vi "P541 Test.vi"() -> ()   [LabVIEW 2014]
uses:
  Controls/StageStates.ctl
panel:
  out "x-y":u32
  in  "Abort":refnum<vi>
  in  "stop":bool
  out "Monitor":cluster{"Numeric":dbl}(graph) caption="N664"
  in  "Sample Z - P541":T1={"Step Up"=FALSE, "Step Down"=FALSE, "Z Position"=0.0, "Step Size (um)"=1.0}
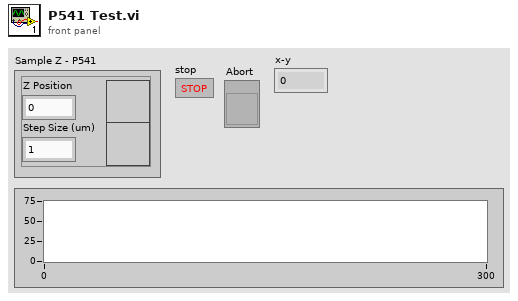
[diagram p1: front panel]
types:
  T1 = cluster{"Step Up":bool, "Step Down":bool, "Z Position":dbl, "Step Size (um)":dbl}
  T2 = typedef "StageStates.ctl" = enum16{"POSITION", "MVR", "MOVE", "HALT", "ONTARGET", "ERROR", "EXIT", "HOME", "ZEROPOS", "NANOPOS", "QUIT", "ANALOG"}
  T3 = cluster{"Step Up":bool, "Step Down":bool, "Z Position":bool, "Step Size (um)":bool}
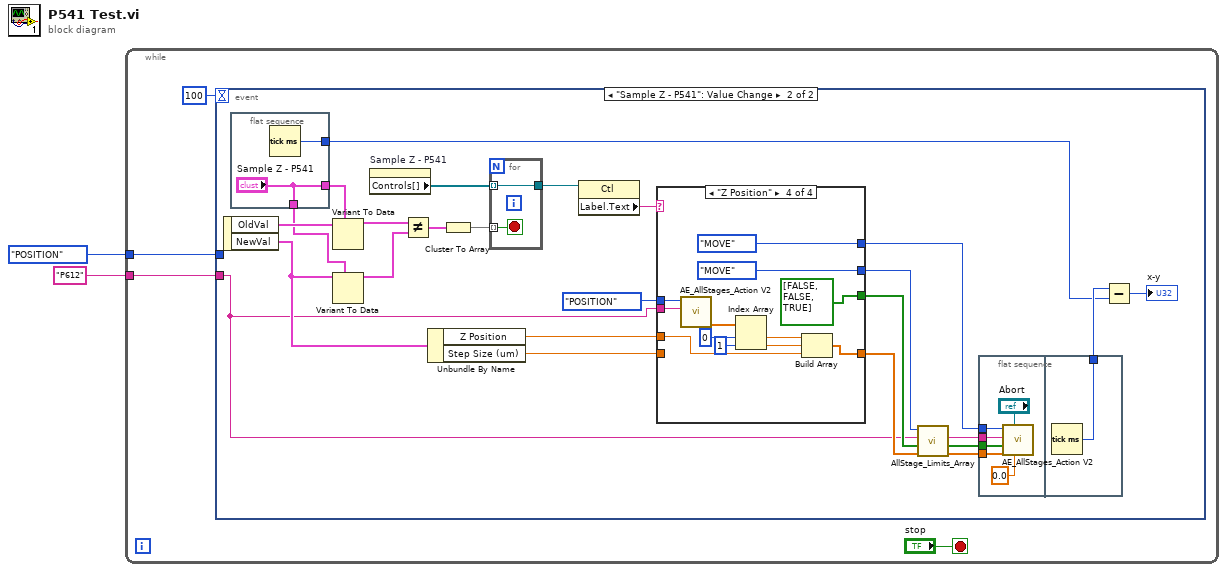
[diagram p0: block diagram]
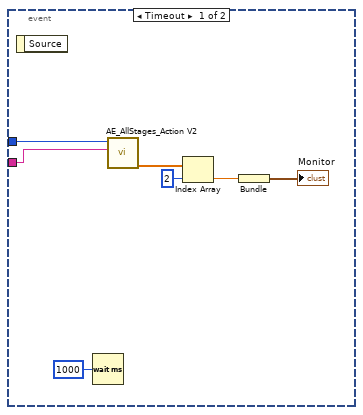
[diagram p2: hidden frame]
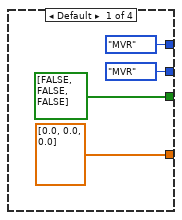
[diagram p3: hidden frame]
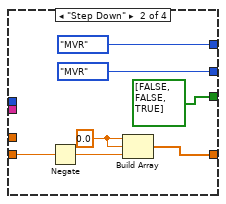
[diagram p4: hidden frame]
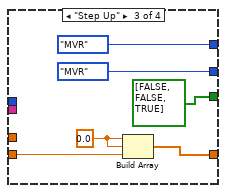
[diagram p5: hidden frame]
diagram:
  n1 = while {
    tunnel: StageStates."POSITION" ("Action") -> [w5]
    tunnel: "P612" ("Stage ID") -> [w4]
    stop <- "stop" stop-if-true
    n2 = event shown="[1] \"Sample Z - P541\": Value Change" {
      selector: _ -> [_ _]
      dyn-events: _ -> [_ _]
      timeout: 100 -> [_ _]
      tunnel: w5 -> [w12 _]
      tunnel: w4 -> [w11 w18]
      event Timeout {
        n3 = event-data() -> ()  [unwired: 1 in, 1 out]
        n4 = Wait (ms)(milliseconds to wait=u32 1000) -> ()  [unwired: 1 out]
        n5 = call "AE_AllStages_Action V2.vi"("Stage ID"=w11, "Action"=w12) -> ("Position Out"=w10:dbl[])  [unwired: 7 in, 2 out]
        n6 = Index Array(array=w10, index=2) -> (element=w8:dbl)
        n7 = Bundle("Numeric"=w8) -> (→"Monitor":cluster{"Numeric":dbl})  [unwired: 1 in]
      }
      event "Sample Z - P541": Value Change {
        n8 = event-data() -> ("OldVal"=w38:T1, "NewVal"=w29:T1)  [unwired: 1 in]
        n9 = flat-sequence {
          tunnel: ["Sample Z - P541"] -> w36
          tunnel: ["Sample Z - P541"] -> w17
          tunnel: [w39] -> w15
          frame #0 {
            n10 = Tick Count (ms)() -> (millisecond timer value=w39:u32)
          }
        }
        n11 = Variant To Data(type=w36, Variant=w38) -> (data=w37:T1)  [unwired: 1 in, 1 out]
        n12 = Variant To Data(type=w17, Variant=w29) -> (data=w35:T1)  [unwired: 1 in, 1 out]
        n13 = property on="Sample Z - P541" class="Clust"() -> ("Controls[]"=w32:refnum<vi>[])  [unwired: 2 in, 2 out]
        n14 = Not Equal?(x=w37, y=w35) -> (x != y?=w34:T3)
        n15 = Unbundle By Name(w29) -> ("Z Position"=w27:dbl, "Step Size (um)"=w28:dbl)
        n16 = Cluster To Array(cluster=w34) -> (array=w33:bool[])
        n17 = for {
          tunnel: w33 -> [w77] mode=indexing
          tunnel: w32 -> [w78] mode=indexing
          tunnel: [w78] -> w31
          stop <- w77 stop-if-true
        }
        n18 = property class="Ctl"(reference=w31) -> ("Label.Text"=w30:string)  [unwired: 1 in, 2 out]
        n19 = case shown="\"Z Position\"" w30 {
          tunnel: w28 -> [_ w55 w59 _]
          tunnel: [StageStates."MVR" ("Action") StageStates."MVR" ("Action") StageStates."MVR" ("Action") StageStates."MOVE" ("Action")] -> w25
          tunnel: [enum16{"MOVE", "MVR"}."MVR" ("MOVE/MVR") enum16{"MOVE", "MVR"}."MVR" ("MOVE/MVR") enum16{"MOVE", "MVR"}."MVR" ("MOVE/MVR") enum16{"MOVE", "MVR"}."MOVE" ("MOVE/MVR")] -> w26
          tunnel: [bool[] [FALSE, FALSE, FALSE] bool[] [FALSE, FALSE, TRUE] bool[] [FALSE, FALSE, TRUE] bool[] [FALSE, FALSE, TRUE]] -> w20
          tunnel: [dbl[] [0.0, 0.0, 0.0] w54 w61 w73] -> w21
          tunnel: w27 -> [_ _ _ w65]
          tunnel: StageStates."POSITION" ("Action") -> [_ _ _ w72]
          tunnel: w18 -> [_ _ _ w71]
          frame Default {
          }
          frame "Step Down" {
            w52 = 0.0 ("element")
            n20 = Negate(x=w55) -> (-x=w53:dbl)
            n21 = Build Array(w52, w52, w53) -> (w54:dbl[])
          }
          frame "Step Up" {
            w60 = 0.0 ("element")
            n22 = Build Array(w60, w60, w59) -> (w61:dbl[])
          }
          frame "Z Position" {
            n23 = call "AE_AllStages_Action V2.vi"("Stage ID"=w71, "Action"=w72) -> ("Position Out"=w70:dbl[])  [unwired: 7 in, 2 out]
            n24 = Index Array(array=w70, index #1=0 ("index"), index #2=1 ("index")) -> (element #1=w67:dbl, element #2=w66:dbl)
            n25 = Build Array(w67, w66, w65) -> (w73:dbl[])
          }
        }
        n26 = call "AllStage_Limits_Array.vi"("Step(um)/Position(units)"=w21, "Axis"=w20, "Stage ID"=w18, "MOVE/MVR"=w26) -> ("Positions"=w22:dbl[], "Boolean Array"=w23:bool[], "Stage ID"=w24:string)  [unwired: 4 in, 1 out]
        n27 = flat-sequence {
          tunnel: w25 -> [w46]
          tunnel: w24 -> [w45]
          tunnel: w23 -> [w44]
          tunnel: w22 -> [w43]
          tunnel: [w47] -> w16
          frame #0 {
            n28 = call "AE_AllStages_Action V2.vi"("Velocity"=0.0, "Abort"="Abort", "Positions"=w43, "Axis"=w44, "Stage ID"=w45, "Action"=w46) -> ()  [unwired: 3 in, 3 out]
          }
          frame #1 {
            n29 = Tick Count (ms)() -> (millisecond timer value=w47:u32)
          }
        }
        n30 = Subtract(x=w16, y=w15) -> (x-y=→"x-y":u32)
      }
    }
  }
